vi "Read (Waveform)Metodo.vi"(8 "error in (no error)":errorcluster, 9 "Timeout (10000 ms)":u32=10000, 10 "Source (0: Channel 1)":u16(ring) items=["Channel 1", "Channel 2", "Channel 3", "Channel 4", "Math", "Reference A", "Reference B", "Reference C", "Reference D", "FFT"], 11 "Keysight in":refnum<class "Edu-1200.lvclass">) -> (0 "error out":errorcluster, 2 "Waveform Data":waveform(dbl)(graph), 3 "Keysight out":refnum<class "Edu-1200.lvclass">)   [LabVIEW 2020, in "Edu-1200.lvclass"]
uses:
  Edu-1200.lvclass
  Edu-1200.lvclass/Edu-1200.ctl
  <instrlib>/Agilent 2000 3000 X-Series/Agilent 2000 3000 X-Series.lvlib
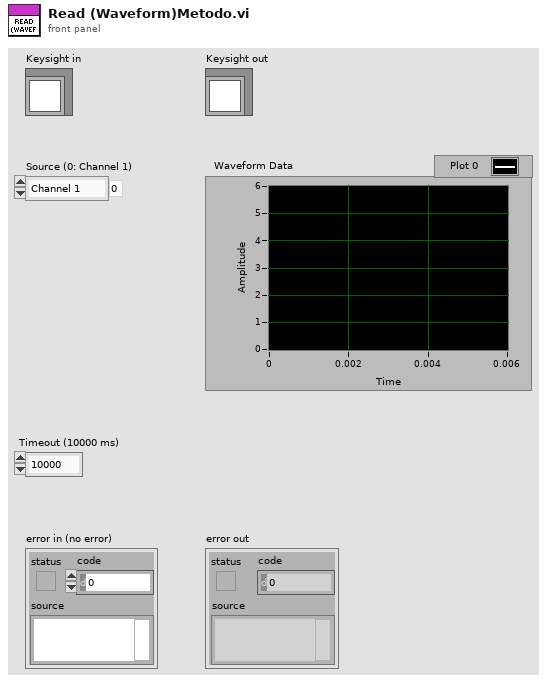
[diagram p1: front panel]
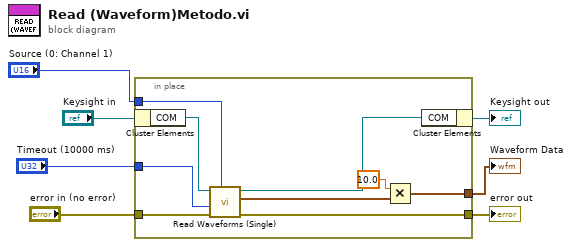
[diagram p0: block diagram]
diagram:
  n1 = in-place {
    in-place-border: [w14] -> w5
    in-place-border: [w9] -> w4
    in-place-border: "error in (no error)" -> [w13]
    in-place-border: "Timeout (10000 ms)" -> [w12]
    in-place-border: "Source (0: Channel 1)" -> [w8]
    n2 = in-place-cluster #1("Keysight in") -> ("COM"=w16:refnum<visa-resource-name>)
    n3 = call <instrlib>:"Read Waveforms (Single).vi"("Bind Source Channel (2: None)"=w8, "error in (no error)"=w13, "Timeout (10000 ms)"=w12, "VISA resource name"=w16) -> ("error out"=w14:errorcluster, "Waveform Data"=w11:waveform(dbl), "VISA resource name out"=w15:refnum<visa-resource-name>)  [unwired: 1 in, 4 out]
    n4 = Multiply(x=10.0, y=w11) -> (x*y=w9:waveform(dbl))
    n5 = in-place-cluster #1("COM"=w15) -> (→"Keysight out":refnum<class "Edu-1200.lvclass">)
  }
  "Waveform Data" <- w4
  "error out" <- w5
